vi "Query Overvolt Protection State.vi"(8 "error in (no error)":errorcluster, 11 "VISA resource name":refnum<visa-resource-name>) -> (0 "error out":errorcluster, 2 "Over Voltage Protection":bool, 3 "VISA resource name out":refnum<visa-resource-name>)   [LabVIEW 2018, in "Agilent E364X Series.lvlib"]
doc: "This VI returns whether the power supply is in a Over Voltage state.\n\nAn over-voltage condition occurs when the output voltage is equal to or greater than the value of the OVP value set and if OVP is currently enabled.\n\n\nWhen an over-voltage condition occurs, the power supply's output protection disables the output. If the power supply is in an over-voltage, it does not produce power until the output protection is reset. The hpe364xa Reset Overvolt Protection VI resets the overvolt protection. Once the overvolt protection is reset, the power supply resumes generating a power signal."
uses:
  Agilent E364X Series.lvlib
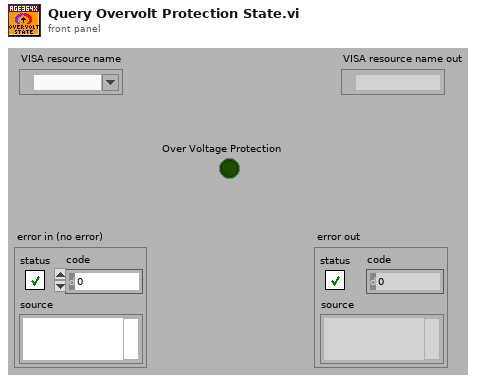
[diagram p1: front panel]
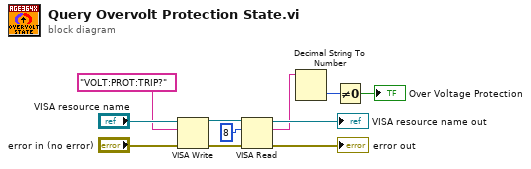
[diagram p0: block diagram]
diagram:
  n1 = VISA Write(VISA resource name="VISA resource name", write buffer="VOLT:PROT:TRIP?", error in (no error)="error in (no error)") -> (VISA resource name out=w2:refnum<visa-resource-name>, error out=w1:errorcluster)  [unwired: 1 out]
  n2 = VISA Read(VISA resource name=w2, byte count=u32 8, error in (no error)=w1) -> (VISA resource name out=→"VISA resource name out":refnum<visa-resource-name>, read buffer=w5:string, error out=→"error out":errorcluster)  [unwired: 1 out]
  n3 = Decimal String To Number(string=w5) -> (number=w4:i32)  [unwired: 2 in, 1 out]
  n4 = Not Equal To 0?(x=w4) -> (x != 0?=→"Over Voltage Protection":bool)
